vi "Assert 2D Array wired to 1D Array Type.vi"   [LabVIEW 2017]
uses:
  03b42b43-3291-44c0-b98d-19a6d8e75211.vi
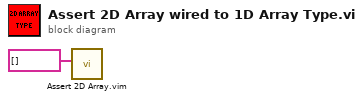
[diagram p0: block diagram]
diagram:
  n1 = call "Assert 2D Array.vim"("Array in"=string[] []) -> ()  [unwired: 10 in, 1 out]
